vi "JAPCtiming.vi"(8 "error in (no error)":errorcluster, 11 "URLs":string[](array[string])) -> (0 "error out":errorcluster, 1 "Values in mbar":dbl[](array[numeric]), 3 "Time in ms":dbl[](array[numeric]))   [LabVIEW 2014]
uses:
  <userlib>/_RADE/RIO/JAPC/classes/JGet/openJAPCGet.vi
  <userlib>/_RADE/RIO/JAPC/classes/JGet/JAPCGet.vi
  <userlib>/_RADE/RIO/JAPC/classes/JGet/JGet.lvclass
panel:
  out "Data 2":variant
  out "element":string
  out "Loop":i32
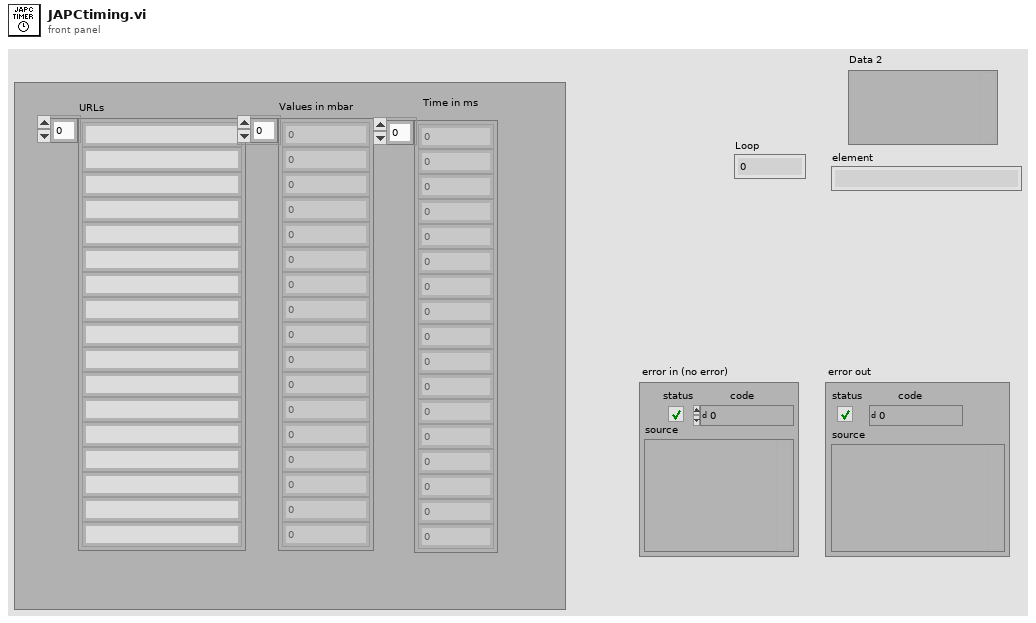
[diagram p1: front panel]
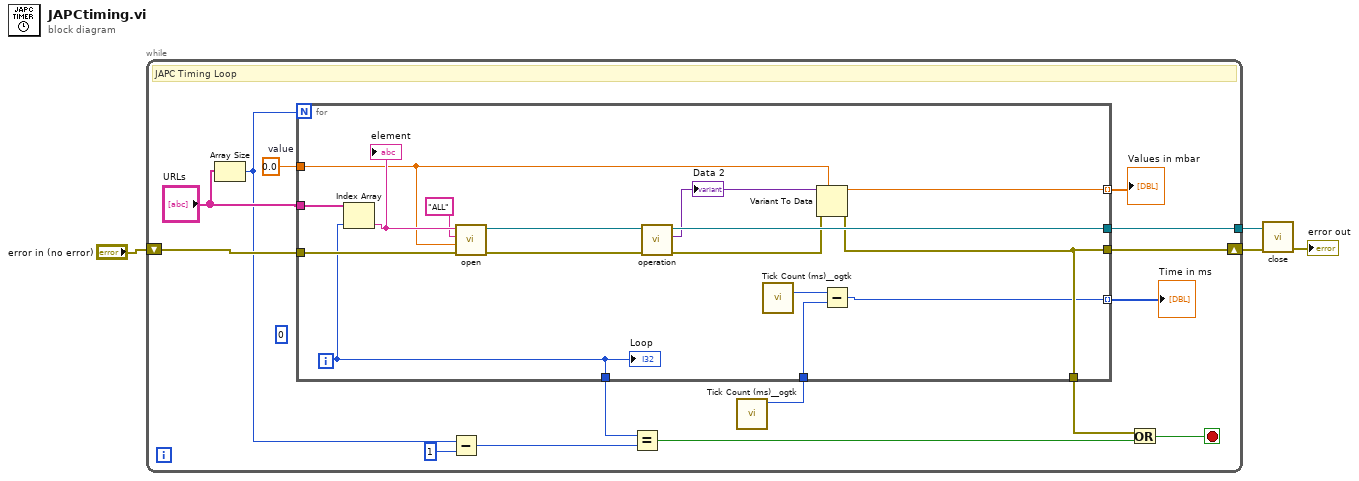
[diagram p0: block diagram]
diagram:
  n1 = while {
    tunnel: [w16] -> w2
    shift-right: [w15] -> w1
    shift-left: "error in (no error)" -> [w17]
    stop <- w14 stop-if-true
    (unwired) u32 0
    w13 = 0.0  # value
    # "JAPC Timing Loop"
    n2 = Array Size(array="URLs") -> (size(s)=w5:i32)
    n3 = Subtract(x=w5, y=1) -> (x-y=w10:i32)
    n4 = call <userlib>:"Tick Count (ms)__ogtk.vi"() -> ("millisecond timer value"=w7:u32)  [unwired: 10 in, 1 out]
    n5 = for {
      N: w5 -> [_]
      tunnel: w13 -> [w20]
      tunnel: [w28] -> w19
      tunnel: [w35] -> w18 mode=indexing
      tunnel: w17 -> [w33]
      tunnel: "URLs" -> [w31]
      tunnel: [w29] -> w16
      tunnel: [w28] -> w15
      tunnel: [w21] -> w12
      tunnel: [w22] -> w8 mode=indexing
      tunnel: w7 -> [w23]
      i -> [w21]
      n6 = Index Array(array=w31, index=w21) -> (element=w30:string)
      "element" <- w30
      n7 = call-poly <userlib>:"open.vi"("error in (no error)"=w33, "Data type"=w20, "Cycle"="ALL", "URL"=w30) -> ("error out"=w34:errorcluster, "Object out"=w32:refnum<class "JGet.lvclass">)  [unwired: 6 in]
      n8 = call-poly <userlib>:"operation.vi"("error in (no error)"=w34, "Object in"=w32) -> ("error out"=w26:errorcluster, "Data"=w25:variant, "Object out"=w29:refnum<class "JGet.lvclass">)  [unwired: 5 in, 2 out]
      "Data 2" <- w25
      n9 = call <userlib>:"Tick Count (ms)__ogtk.vi"() -> ("millisecond timer value"=w24:u32)  [unwired: 10 in, 1 out]
      n10 = Variant To Data(error in=w26, type=w20, Variant=w25) -> (data=w35:dbl, error out=w28:errorcluster)
      n11 = Subtract(x=w24, y=w23) -> (x-y=w22:u32)
      "Loop" <- w21
    }
    "Values in mbar" <- w18
    "Time in ms" <- w8
    n12 = Equal?(x=w12, y=w10) -> (x = y?=w11:bool)
    n13 = Or(x=w19, y=w11) -> (x .or. y?=w14:bool)
  }
  n14 = call-dynamic "close.vi"("error in (no error)"=w1, "Object in"=w2) -> ("error out"=→"error out":errorcluster)  [unwired: 9 in]
